vi "Thermocouple.vi"   [LabVIEW 2018]
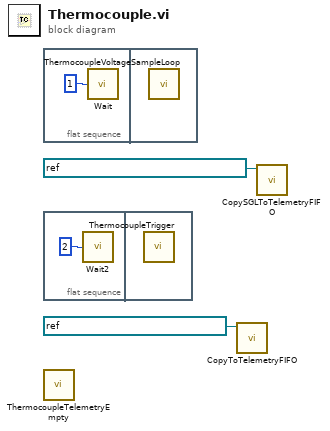
[diagram p0: block diagram]
diagram:
  n1 = flat-sequence {
    frame #0 {
      n2 = call "Wait"("Count(mSec)"=u8 1) -> ()  [unwired: 1 out]
    }
    frame #1 {
      n3 = call "ThermocoupleVoltageSampleLoop.vi"() -> ()  [unwired: 12 in]
    }
  }
  n4 = flat-sequence {
    frame #0 {
      n5 = call "Wait2"("Count(mSec)"=u8 2) -> ()  [unwired: 1 out]
    }
    frame #1 {
      n6 = call "ThermocoupleTrigger.vi"() -> ()  [unwired: 12 in]
    }
  }
  n7 = call "ThermocoupleTelemetryEmpty.vi"() -> ()  [unwired: 12 in]
  n8 = call "CopyToTelemetryFIFO.vi"("SourceFIFO"=refnum<k21> "ThermocoupleTelemetryFIFO") -> ()  [unwired: 11 in]
  n9 = call "CopySGLToTelemetryFIFO.vi"("SourceFIFO"=refnum<k21> "ThermocoupleTelemetrySGLFIFO") -> ()  [unwired: 11 in]
